vi "GoToBallPlacementPositionSkill.vi"(8 "error in (no error)":errorcluster, 9 "Game":refnum<class "Game.lvclass">, 10 "Robot":refnum<class "Robot.lvclass">, 11 "GoToBallPlacementPositionSkill in":refnum<class "GoToBallPlacementPositionSkill.lvclass">) -> (0 "error out":errorcluster, 1 "robotPositionedToReceiveBall":bool, 2 "Robot out":refnum<class "Robot.lvclass">, 3 "GoToBallPlacementPositionSkill out":refnum<class "GoToBallPlacementPositionSkill.lvclass">)   [LabVIEW 2021, in "GoToBallPlacementPositionSkill.lvclass"]
uses:
  GoToBallPlacementPositionSkill.lvclass
  Robot_class/Robot.lvclass
  D:/RoboIme/horie/SSL_AI/Object_class/Object.lvclass
  Game_class/Game.lvclass
  Game_class/Game.lvclass/Game.ctl
  Object_class/Object.lvclass/Object.ctl
  Robot_class/Robot.lvclass/Robot.ctl
  <vilib>/Analysis/baseanly.llb/Unit Vector (DBL).vi
  <vilib>/Analysis/coordinate.llb/Wrap Angle (scalar).vi
  Object_class/Read position(x,y).vi
  Robot_class/Read orientation.vi
  Game_class/Read BallRef.vi
  Game_class/Read Referee.vi
  Robot_class/Write dest_x.vi
  Robot_class/Write dest_y.vi
  Robot_class/Write dest_orientation.vi
  Ball_class/Ball.lvclass
  Referee_class/Referee.lvclass
  <vilib>/Analysis/NI_AALBase.lvlib
  Utilities_class/Utilities.lvclass
  <vilib>/Analysis/NI_AAL_Angle.lvlib
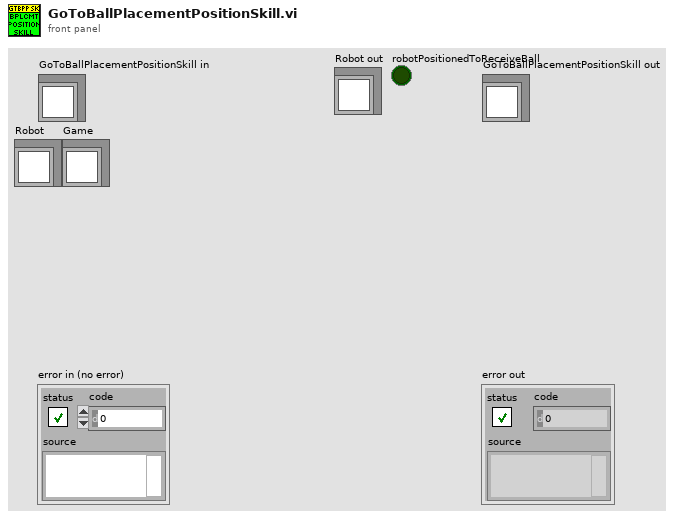
[diagram p1: front panel]
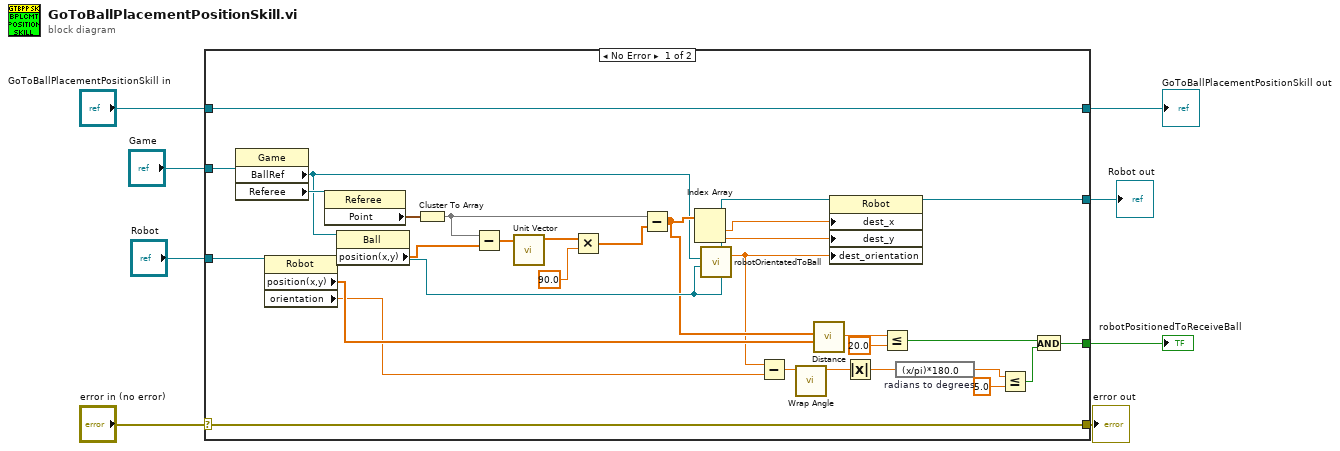
[diagram p0: block diagram]
diagram:
  n1 = case shown="No Error" "error in (no error)" {
    selector: "error in (no error)" -> [w38 w41]
    tunnel: [w38 w41] -> w7
    tunnel: [w39 w40] -> w5
    tunnel: "GoToBallPlacementPositionSkill in" -> [w39 w40]
    tunnel: "Game" -> [w37 _]
    tunnel: "Robot" -> [w34 _]
    tunnel: [w25 _] -> w2
    tunnel: [w11 _] -> w1
    frame No Error {
      n2 = property class="Game"(reference=w37) -> ("BallRef"=w10:refnum<class "Ball.lvclass">, "Referee"=w36:refnum<class "Referee.lvclass">)  [unwired: 1 in, 2 out]
      n3 = property class="Robot"(reference=w34) -> (reference out=w26:refnum<class "Robot.lvclass">, "position(x,y)"=w24:dbl[], "orientation"=w18:dbl)  [unwired: 1 in, 1 out]
      n4 = property class="Referee"(reference=w36) -> ("Point"=w35:cluster{"x":sgl, "y":sgl})  [unwired: 1 in, 2 out]
      n5 = property class="Ball"(reference=w10) -> ("position(x,y)"=w9:dbl[])  [unwired: 1 in, 2 out]
      n6 = Cluster To Array(cluster=w35) -> (array=w33:sgl[])
      n7 = Subtract(x=w33, y=w9) -> (x-y=w32:dbl[])
      n8 = call-poly <vilib>:"Unit Vector.vi"("Input Vector"=w32) -> ("Unit Vector"=w31:dbl[])  [unwired: 8 in, 2 out]
      n9 = Multiply(x=w31, y=90.0) -> (x*y=w29:dbl[])
      n10 = Subtract(x=w33, y=w29) -> (x-y=w23:dbl[])
      n11 = Index Array(array=w23) -> (element #1=w28:dbl, element #2=w27:dbl)  [unwired: 2 in]
      n12 = call "robotOrientatedToBall.vi"("Robot"=w26, "BallRef"=w10) -> ("Orientation"=w19:dbl)  [unwired: 7 in, 2 out]
      n13 = Subtract(x=w19, y=w18) -> (x-y=w17:dbl)
      n14 = call-poly <vilib>:"Wrap Angle.vi"("angle in"=w17) -> ("angle out"=w16:dbl)  [unwired: 9 in, 1 out]
      n15 = call "Distance.vi"("P1"=w24, "P2"=w23) -> ("Distance"=w22:dbl)  [unwired: 7 in, 2 out]
      n16 = property class="Robot"(reference=w26, "dest_x"=w28, "dest_y"=w27, "dest_orientation"=w19) -> (reference out=w25:refnum<class "Robot.lvclass">)  [unwired: 1 in, 1 out]
      n17 = Absolute Value(x=w16) -> (abs(x)=w15:dbl)
      n18 = Less Or Equal?(x=w22, y=20.0) -> (x <= y?=w20:bool)
      n19 = expression code="(x/pi)*180.0" "radians to degrees"(w15) -> (w14:dbl)
      n20 = Less Or Equal?(x=w14, y=5.0) -> (x <= y?=w12:bool)
      n21 = And(x=w20, y=w12) -> (x .and. y?=w11:bool)
    }
    frame Error {
    }
  }
  "error out" <- w7
  "GoToBallPlacementPositionSkill out" <- w5
  "Robot out" <- w2
  "robotPositionedToReceiveBall" <- w1
